vi "Teleop_DriveFwd.vi"(10 "Joy_R_Buttons":bool[](array[boolean]), 11 "Joy_R_Axes":dbl[](array[numeric])) -> (1 "Deadband FWD":bool=TRUE, 3 "drive output":dbl)   [LabVIEW 2017]
uses:
  TypeDefs/joybuttons.ctl
  TypeDefs/joyaxes.ctl
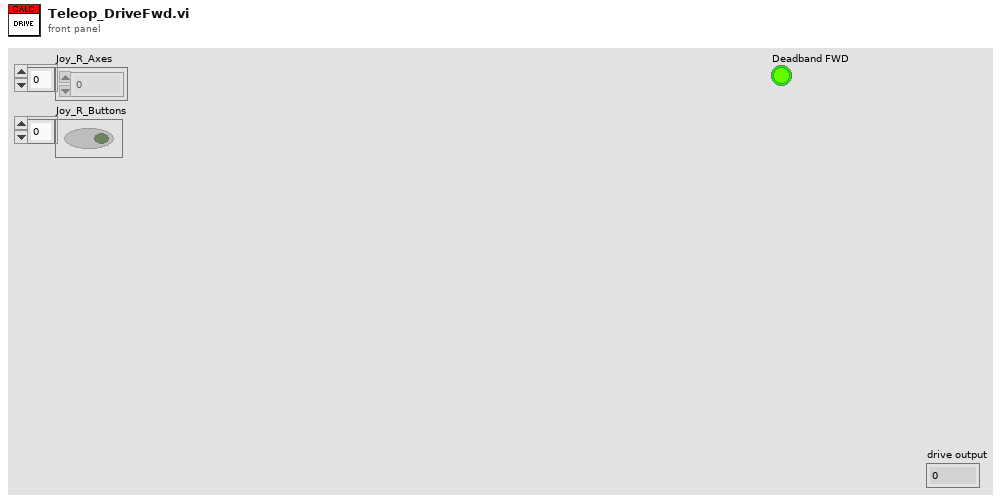
[diagram p1: front panel]
types:
  T1 = typedef "joyaxes.ctl" = enum16{"x axis", "y axis", "twist", "throttle"}
  T2 = typedef "joybuttons.ctl" = enum16{"Trigger", "Thumb", "Top3", "Top4", "Top5", "Top6", "Bottom7", "Bottom8", "Bottom9", "Bottom10", "Bottom11", "Bottom12", ""}
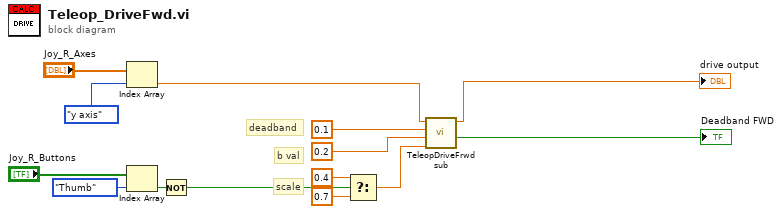
[diagram p0: block diagram]
diagram:
  # "scale"
  # "b val"
  # "deadband"
  n1 = Index Array(array="Joy_R_Axes", index=joyaxes."y axis" ("Enum")) -> (element=w2:dbl)
  n2 = Index Array(array="Joy_R_Buttons", index=joybuttons."Thumb" ("Enum")) -> (element=w13:bool)
  n3 = Not(x=w13) -> (.not. x?=w9:bool)
  n4 = Select(t=0.4, s=w9, f=0.7) -> (s? t:f=w5:dbl)
  n5 = call "TeleopDriveFrwdsub.vi"("SCALE"=w5, "B VALUE"=0.2, "Deadband X value"=0.1, "Drive"=w2) -> ("Deadband FWD"=→"Deadband FWD":bool, "Drive Output"=→"drive output":dbl)  [unwired: 6 in]
